vi "力特性.vi"(8 "error in (no error)":errorcluster caption="错误输入（无错误）", 11 "信号数据":dbl[][](array[numeric])) -> (0 "error out":errorcluster caption="错误输出")   [LabVIEW 2015, in "Logging.lvlib"]
uses:
  Logging.lvlib
panel:
  out "偏差角度":dbl format="%0.2f"
  in  "推力选择":dbl=136.0
  out "C+5MPa扭矩右":dbl
  out "C+5MPa扭矩左":dbl
  out "C+0.5MPa扭矩右":dbl
  out "DE扭矩差右":dbl
  out "C+0.5MPa扭矩左":dbl
  out "DE扭矩差左":dbl
  out "8MPa扭矩右":dbl
  out "5MPa扭矩右":dbl
  out "3MPa扭矩右":dbl
  out "8MPa扭矩左":dbl
  out "5MPa扭矩左":dbl
  out "3MPa扭矩左":dbl
  out "最大扭矩右":dbl
  out "136KG推力右扭矩":dbl
  out "回正率":dbl
  out "不灵敏区扭矩":dbl
  out "曲线对称性":dbl
  out "最大扭矩左":dbl
  out "136KG推力左扭矩":dbl
  out "左右扭矩差值":dbl
  out "5MPa对称性":dbl
  out "1MPa对称性":dbl
  in  "取消按钮":bool
  in  "确定按钮":bool
  # "力特性测量结果"
  # "KG"
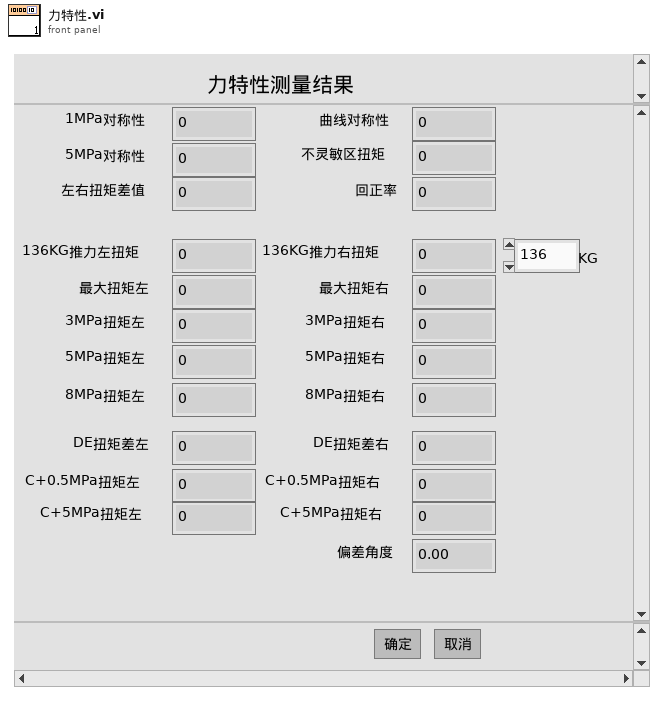
[diagram p1: front panel]
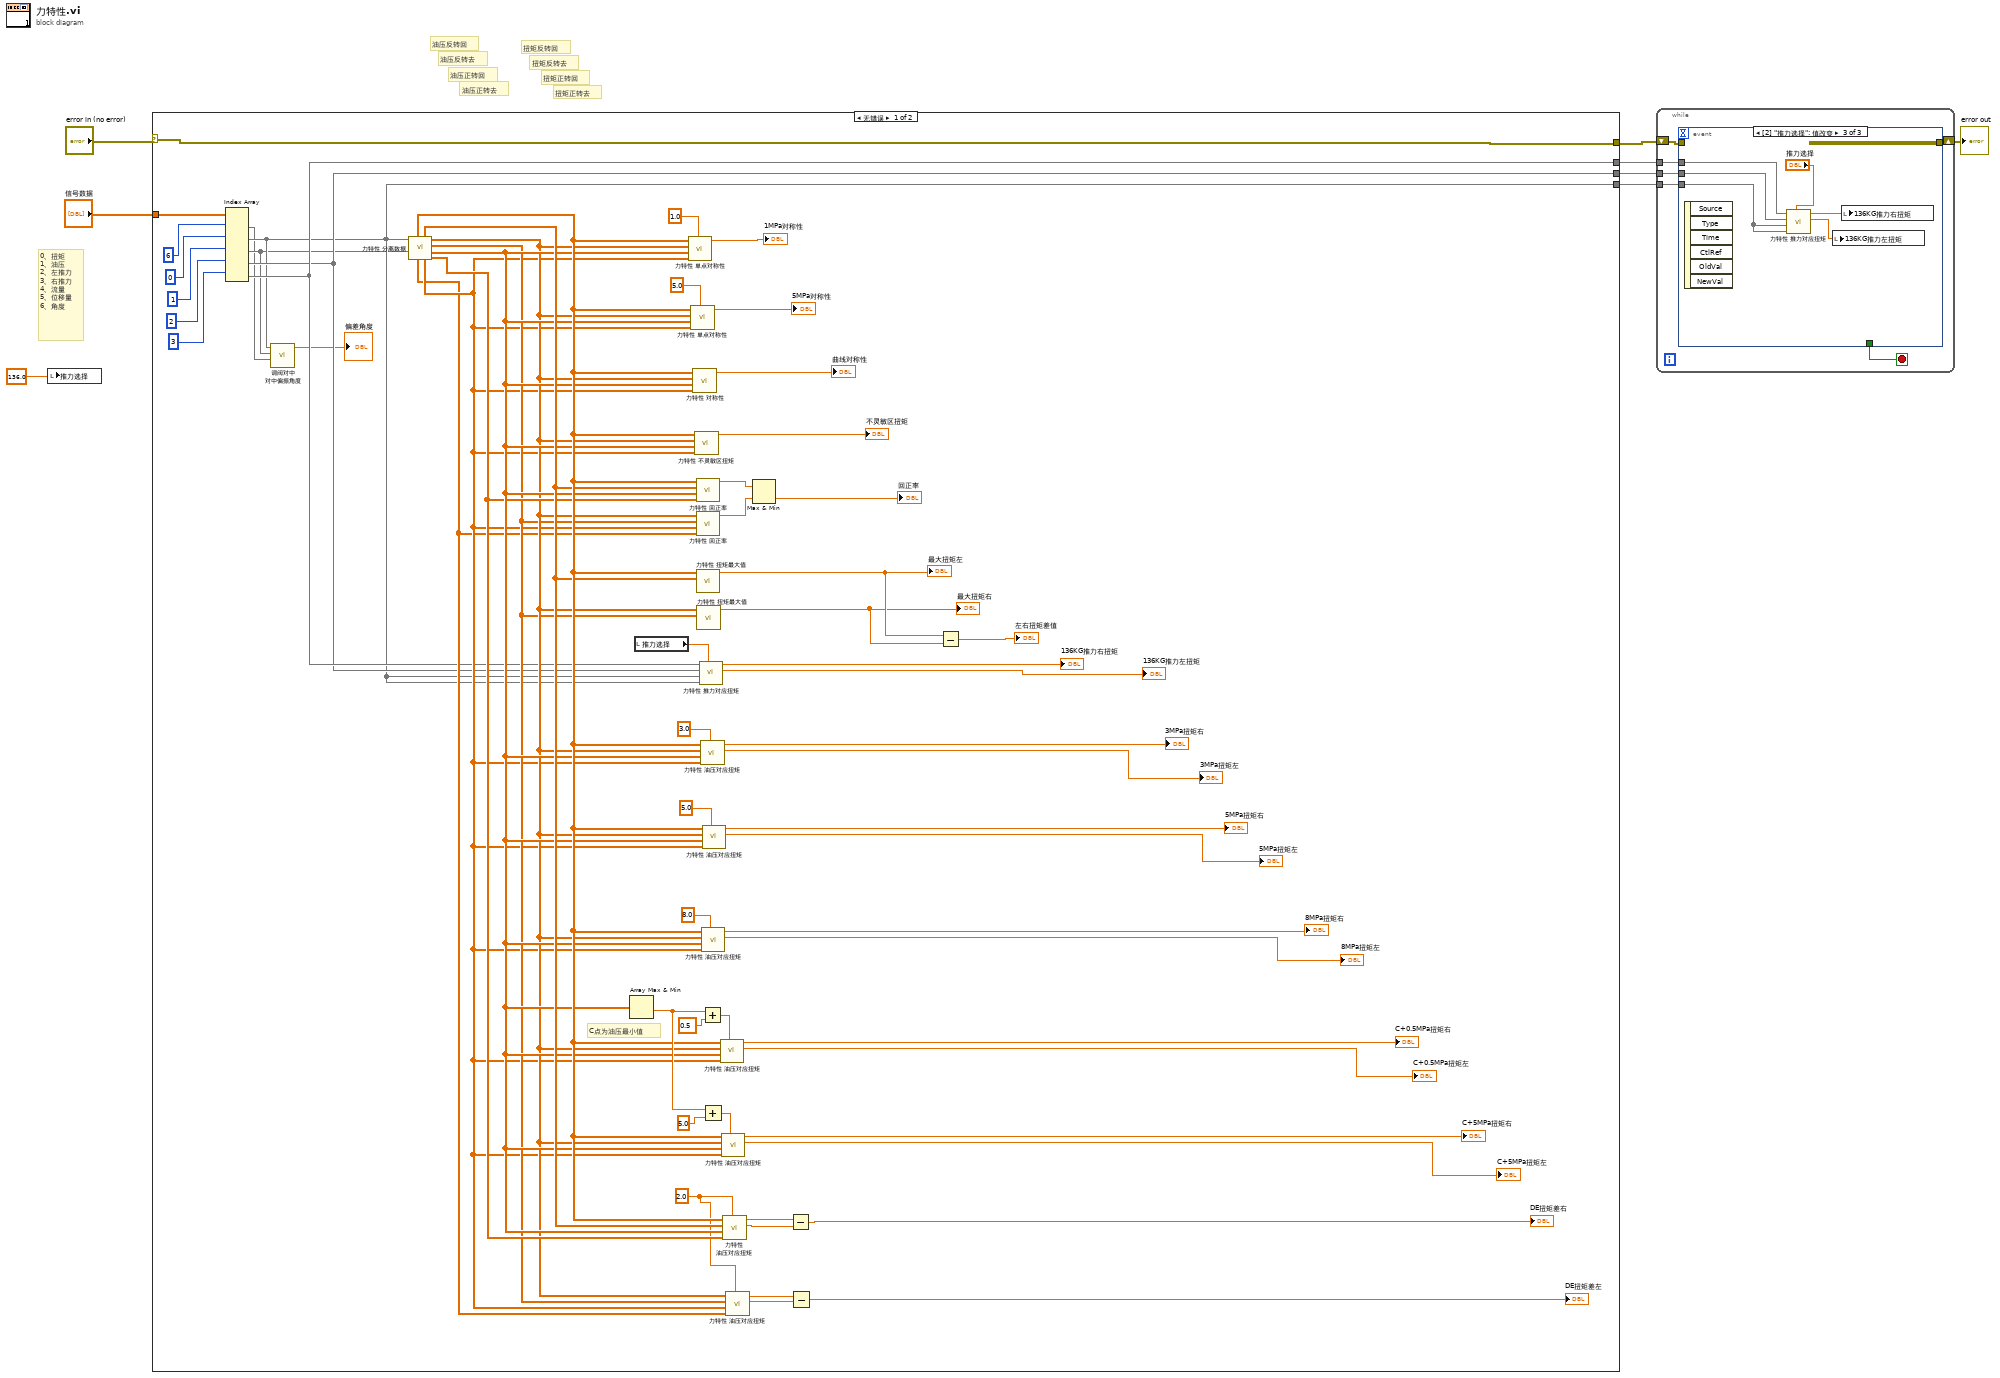
[diagram p0: block diagram]
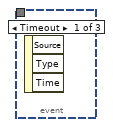
[diagram p2: hidden frame]
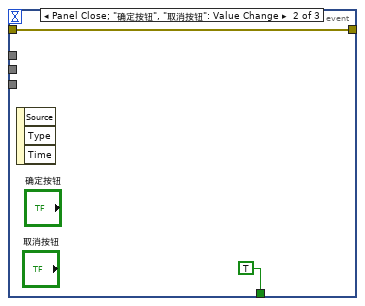
[diagram p3: hidden frame]
diagram:
  # "扭矩正转去"
  # "扭矩正转回"
  # "扭矩反转去"
  # "扭矩反转回"
  # "油压正转去"
  # "油压正转回"
  # "油压反转去"
  # "油压反转回"
  # "0、扭矩\n1、油压\n2、左推力\n3、右推力\n4、流量\n5、位移量\n6、角度"
  n1 = local write "推力选择"(136.0) -> ()
  n2 = case shown="无错误" "error in (no error)" {
    selector: "error in (no error)" -> [w15 w70]
    tunnel: "信号数据" -> [w69 _]
    tunnel: [w15 w70] -> w5
    tunnel: [w14 _] -> w3
    tunnel: [w13 _] -> w2
    tunnel: [w12 _] -> w1
    frame No Error {
      w22 = 2.0
      # "C点为油压最小值"
      n3 = Index Array(array=w69, index (row) #1=6 ("禁用的索引 (列)"), index (row) #2=0 ("索引 (行)"), index (row) #3=1 ("索引 (行)"), index (row) #4=2 ("索引 (行)"), index (row) #5=3 ("索引 (行)")) -> (element #1=w10:dbl[], element #2=w12:dbl[], element #3=w11:dbl[], element #4=w13:dbl[], element #5=w14:dbl[])  [unwired: 5 in]
      n4 = call "调阀对中 对中偏振角度.vi"("角度"=w10, "油压"=w11, "扭矩"=w12) -> ("偏差角度"=→"偏差角度":dbl)  [unwired: 8 in]
      n5 = call "力特性 分离数据.vi"("油压"=w11, "扭矩"=w12) -> ("油压正转回"=w27:dbl[], "油压正转去"=w28:dbl[], "扭矩反转回"=w25:dbl[], "扭矩反转去"=w26:dbl[], "油压反转去"=w24:dbl[], "扭矩正转回"=w29:dbl[], "油压反转回"=w23:dbl[], "扭矩正转去"=w30:dbl[])  [unwired: 2 in]
      n6 = Array Max & Min(array=w28) -> (min value=w39:dbl)  [unwired: 3 out]
      n7 = local read "推力选择"() -> (w54:dbl)
      n8 = call "力特性 单点对称性.vi"("单点压力"=1.0, "油压B"=w24, "油压A"=w28, "扭矩B"=w26, "扭矩A"=w30) -> ("对称性"=→"1MPa对称性":dbl)  [unwired: 6 in]
      n9 = call "力特性 单点对称性.vi"("单点压力"=5.0, "油压B"=w24, "油压A"=w28, "扭矩B"=w26, "扭矩A"=w30) -> ("对称性"=→"5MPa对称性":dbl)  [unwired: 6 in]
      n10 = call "力特性 对称性.vi"("油压B"=w24, "油压A"=w28, "扭矩B"=w26, "扭矩A"=w30) -> ("对称性"=→"曲线对称性":dbl)  [unwired: 7 in]
      n11 = call "力特性 不灵敏区扭矩.vi"("油压B"=w24, "油压A"=w28, "扭矩B"=w26, "扭矩A"=w30) -> ("不灵敏区扭矩"=→"不灵敏区扭矩":dbl)  [unwired: 7 in]
      n12 = call "力特性 回正率.vi"("油压B"=w27, "油压A"=w28, "扭矩B"=w29, "扭矩A"=w30) -> ("回正率"=w42:dbl)  [unwired: 7 in]
      n13 = call "力特性 回正率.vi"("油压B"=w23, "油压A"=w24, "扭矩B"=w25, "扭矩A"=w26) -> ("回正率"=w41:dbl)  [unwired: 7 in]
      n14 = call "力特性 扭矩最大值.vi"("扭矩回"=w29, "扭矩去"=w30) -> ("扭矩最大值"=w57:dbl)  [unwired: 9 in]
      "最大扭矩左" <- w57
      n15 = call "力特性 扭矩最大值.vi"("扭矩回"=w25, "扭矩去"=w26) -> ("扭矩最大值"=w56:dbl)  [unwired: 9 in]
      "最大扭矩右" <- w56
      n16 = call "力特性 推力对应扭矩.vi"("推力"=w54, "扭矩左"=w12, "扭矩右"=w12, "推力左"=w13, "推力右"=w14) -> ("推力左扭矩"=→"136KG推力左扭矩":dbl, "推力右扭矩"=→"136KG推力右扭矩":dbl)  [unwired: 5 in]
      n17 = call "力特性 油压对应扭矩.vi"("油压"=3.0, "油压B"=w24, "油压A"=w28, "扭矩B"=w26, "扭矩A"=w30) -> ("油压扭矩左"=→"3MPa扭矩左":dbl, "油压扭矩右"=→"3MPa扭矩右":dbl)  [unwired: 5 in]
      n18 = Add(x=w39, y=0.5) -> (x+y=w35:dbl)
      n19 = call "力特性 油压对应扭矩.vi"("油压"=8.0, "油压B"=w24, "油压A"=w28, "扭矩B"=w26, "扭矩A"=w30) -> ("油压扭矩左"=→"8MPa扭矩左":dbl, "油压扭矩右"=→"8MPa扭矩右":dbl)  [unwired: 5 in]
      n20 = Add(x=w39, y=5.0) -> (x+y=w36:dbl)
      n21 = call "力特性 油压对应扭矩.vi"("油压"=5.0, "油压B"=w24, "油压A"=w28, "扭矩B"=w26, "扭矩A"=w30) -> ("油压扭矩左"=→"5MPa扭矩左":dbl, "油压扭矩右"=→"5MPa扭矩右":dbl)  [unwired: 5 in]
      n22 = call "力特性 油压对应扭矩.vi"("油压"=w35, "油压B"=w24, "油压A"=w28, "扭矩B"=w26, "扭矩A"=w30) -> ("油压扭矩左"=→"C+0.5MPa扭矩左":dbl, "油压扭矩右"=→"C+0.5MPa扭矩右":dbl)  [unwired: 5 in]
      n23 = call "力特性 油压对应扭矩.vi"("油压"=w36, "油压B"=w24, "油压A"=w28, "扭矩B"=w26, "扭矩A"=w30) -> ("油压扭矩左"=→"C+5MPa扭矩左":dbl, "油压扭矩右"=→"C+5MPa扭矩右":dbl)  [unwired: 5 in]
      n24 = call "力特性 油压对应扭矩.vi"("油压"=w22, "油压B"=w27, "油压A"=w28, "扭矩B"=w29, "扭矩A"=w30) -> ("油压扭矩左"=w20:dbl, "油压扭矩右"=w21:dbl)  [unwired: 5 in]
      n25 = call "力特性 油压对应扭矩.vi"("油压"=w22, "油压B"=w23, "油压A"=w24, "扭矩B"=w25, "扭矩A"=w26) -> ("油压扭矩左"=w18:dbl, "油压扭矩右"=w19:dbl)  [unwired: 5 in]
      n26 = Max & Min(x=w42, y=w41) -> (min(x,y)=→"回正率":dbl)  [unwired: 1 out]
      n27 = Subtract(x=w21, y=w20) -> (x-y=→"DE扭矩差右":dbl)
      n28 = Subtract(x=w19, y=w18) -> (x-y=→"DE扭矩差左":dbl)
      n29 = Subtract(x=w57, y=w56) -> (x-y=→"左右扭矩差值":dbl)
    }
    frame Error {
    }
  }
  n30 = while {
    shift-right: [w75] -> w4
    shift-left: w5 -> [w76]
    tunnel: w3 -> [w72]
    tunnel: w2 -> [w71]
    tunnel: w1 -> [w73]
    stop <- w74 stop-if-true
    n31 = event shown="[2] \"推力选择\": 值改变" {
      selector: _ -> [_ _ _]
      dyn-events: _ -> [_ _ _]
      timeout: _ -> [_ _ _]
      tunnel: w76 -> [_ w78 _]
      tunnel: [_ w78 _] -> w75
      tunnel: [_ TRUE _] -> w74
      tunnel: w73 -> [_ _ w82]
      tunnel: w72 -> [_ _ w84]
      tunnel: w71 -> [_ _ w83]
      event Timeout {
        n32 = event-data() -> ()  [unwired: 1 in, 3 out]
      }
      event Panel Close; "确定按钮", "取消按钮": Value Change {
        n33 = event-data() -> ()  [unwired: 1 in, 3 out]
      }
      event "推力选择": Value Change {
        n34 = event-data() -> ()  [unwired: 1 in, 6 out]
        n35 = call "力特性 推力对应扭矩.vi"("推力"="推力选择", "扭矩左"=w82, "扭矩右"=w82, "推力左"=w83, "推力右"=w84) -> ("推力左扭矩"=w79:dbl, "推力右扭矩"=w80:dbl)  [unwired: 5 in]
        n36 = local write "136KG推力左扭矩"(w79) -> ()
        n37 = local write "136KG推力右扭矩"(w80) -> ()
      }
    }
  }
  "error out" <- w4
